vi "Phi v2.vi"(6 "Current Hip Angle":dbl, 8 "Hip  Sum":dbl, 9 "Number of samples":dbl, 10 "Feedback In":T1, 11 "Heel Strike?":bool) -> (0 "Feedback Out":T1, 3 "Phi":dbl)   [LabVIEW 2018]
uses:
  Phase Calculator Feedback Cluster.ctl
  <vilib>/ptbypt/NI_PtbyPt.lvlib
panel:
  out "Waveform Chart":dbl(graph)
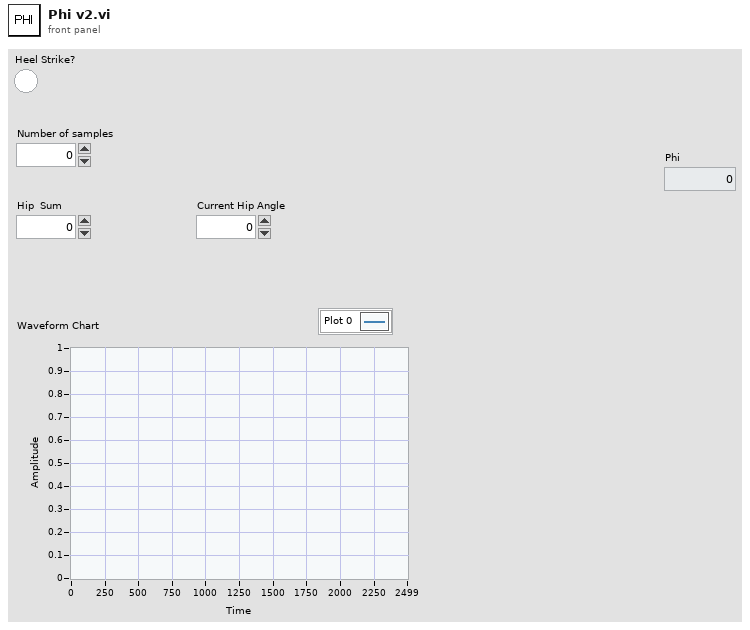
[diagram p1: front panel]
types:
  T1 = typedef "Phase Calculator Feedback Cluster.ctl" = cluster{"k":dbl, "ix0":dbl, "X_max":dbl, "X_min":dbl, "Y_max":dbl, "Y_min":dbl, "Y":dbl, "Hip Sum":dbl, "Num Samples":dbl, "First Heel Strike Done?":bool, "Second Heel Strike Done?":bool, "phi_1":dbl, "phi_end":dbl, "X":dbl}
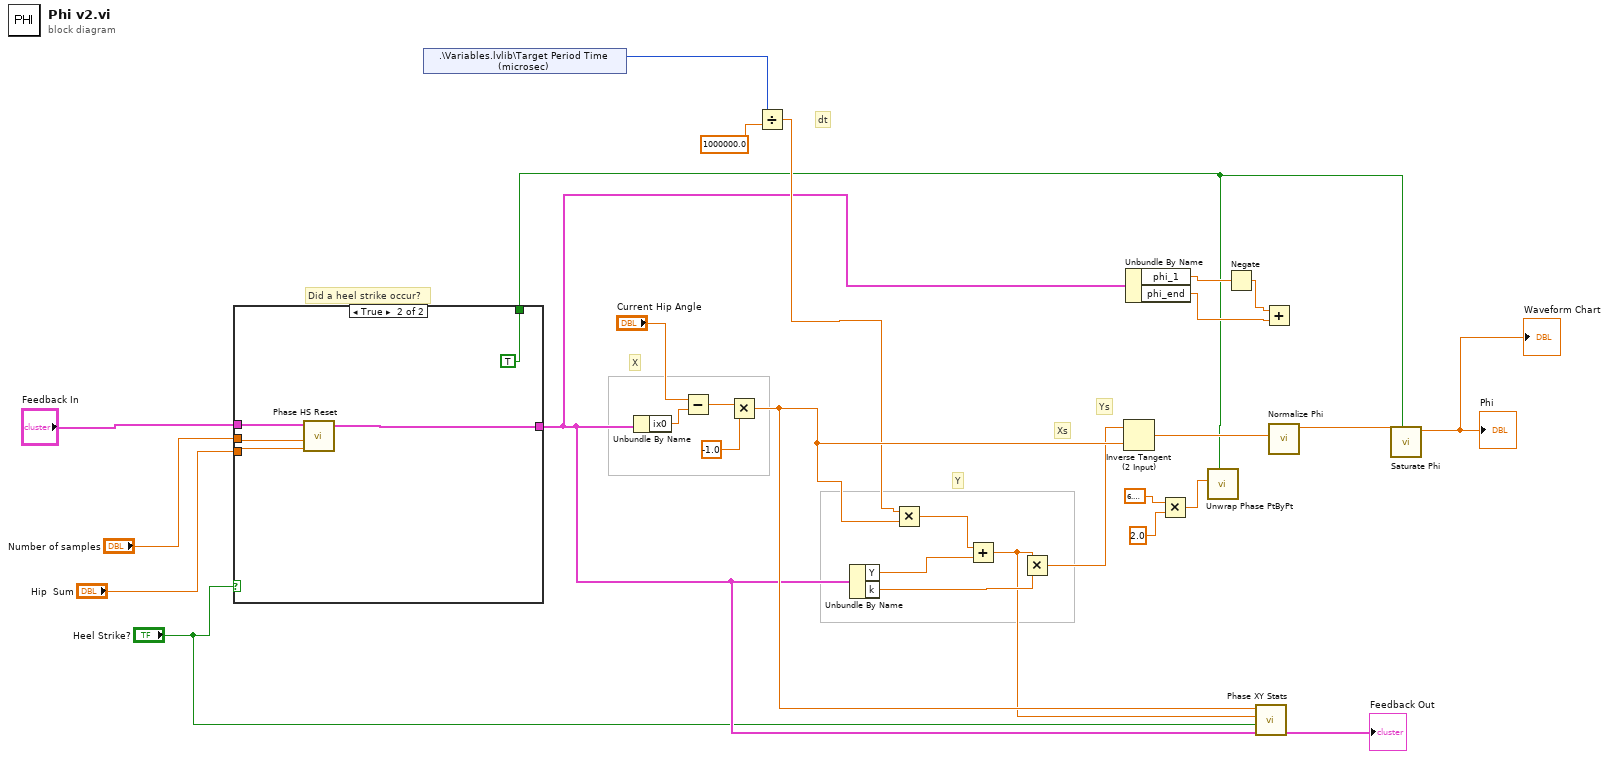
[diagram p0: block diagram]
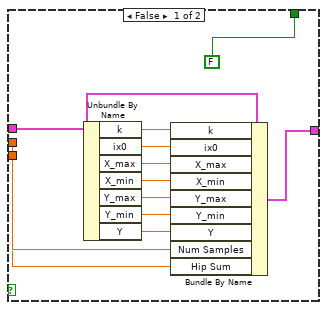
[diagram p2: hidden frame]
diagram:
  # "Xs"
  # "Ys"
  # "Y"
  # "dt"
  # "X"
  # "Did a heel strike occur?"
  n1 = case shown="True" "Heel Strike?" {
    tunnel: "Feedback In" -> [w41 w46]
    tunnel: "Number of samples" -> [w33 w45]
    tunnel: "Hip  Sum" -> [w32 w44]
    tunnel: [w31 w42] -> w9
    tunnel: [FALSE ("initialize") TRUE ("initialize")] -> w2
    frame False {
      n2 = Unbundle By Name(w41) -> ("k"=w40:dbl, "ix0"=w39:dbl, "X_max"=w38:dbl, "X_min"=w37:dbl, "Y_max"=w36:dbl, "Y_min"=w35:dbl, "Y"=w34:dbl)
      n3 = Bundle By Name(cluster=w41, "k"=w40, "ix0"=w39, "X_max"=w38, "X_min"=w37, "Y_max"=w36, "Y_min"=w35, "Y"=w34, "Num Samples"=w33, "Hip Sum"=w32) -> (w31:T1)
    }
    frame True {
      n4 = call "Phase HS Reset.vi"("Hip Sum"=w44, "Number of Samples"=w45, "Feedback In"=w46) -> ("Feedback Out"=w42:T1)  [unwired: 8 in]
    }
  }
  n5 = shared-variable ".\\Variables.lvlib\\Target Period Time (microsec)"() -> (w15:u16)  [unwired: 1 in, 1 out]
  n6 = Unbundle By Name(w9) -> ("ix0"=w26:dbl)
  n7 = Subtract(x="Current Hip Angle", y=w26) -> (x-y=w24:dbl)
  n8 = Multiply(x=w24, y=-1.0) -> (x*y=w18:dbl)
  n9 = Divide(x=w15, y=1000000.0) -> (x/y=w14:dbl)
  n10 = Unbundle By Name(w9) -> ("Y"=w21:dbl, "k"=w20:dbl)
  n11 = Multiply(x=w14, y=w18) -> (x*y=w22:dbl)
  n12 = Add(x=w22, y=w21) -> (x+y=w16:dbl)
  n13 = Multiply(x=w16, y=w20) -> (x*y=w17:dbl)
  n14 = Inverse Tangent (2 Input)(1:w18, 2:w17) -> (0:w4:dbl)
  n15 = Unbundle By Name(w9) -> ("phi_1"=w12:dbl, "phi_end"=w10:dbl)
  n16 = Multiply(x=6.283185307179586, y=2.0) -> (x*y=w6:dbl)
  n17 = call <vilib>:"Unwrap Phase PtByPt.vi"("initialize"=w2, "wrap base"=w6) -> ()  [unwired: 9 in, 1 out]
  n18 = Negate(x=w12) -> (-x=w11:dbl)
  n19 = call "Phase XY Stats.vi"("Feedback In"=w9, "Heel Strike?"="Heel Strike?", "Y"=w16, "X"=w18) -> ("Feedback Out"=→"Feedback Out":T1)  [unwired: 7 in]
  n20 = Add(x=w11, y=w10) -> ()  [unwired: 1 out]
  n21 = call "Normalize Phi.vi"("phi"=w4) -> ("Phi"=w3:dbl)  [unwired: 10 in]
  n22 = call "Saturate Phi.vi"("HS?"=w2, "Phi In"=w3) -> ("Phi Out"=→"Phi" →"Waveform Chart":dbl)  [unwired: 9 in]
